vi "PutBool.vi"(8 "error in (no error)":errorcluster, 10 "Boolean":bool, 11 "MsgPackSerializer in":refnum<class "MsgPackSerializer.lvclass">) -> (0 "error out":errorcluster, 3 "MsgPackSerializer out":refnum<class "MsgPackSerializer.lvclass">)   [LabVIEW 2015, in "MsgPackSerializer.lvclass"]
uses:
  MsgPackSerializer.lvclass
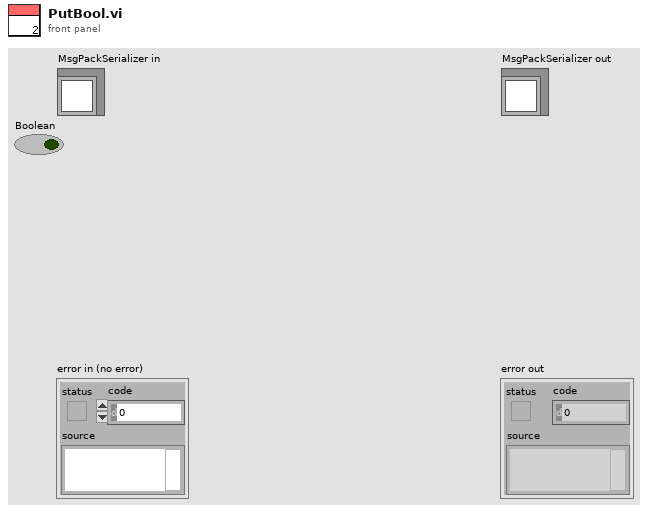
[diagram p1: front panel]
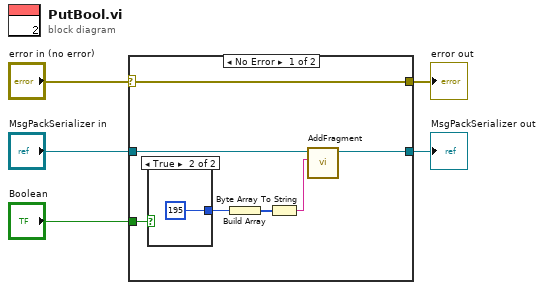
[diagram p0: block diagram]
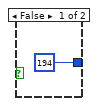
[diagram p2: hidden frame]
diagram:
  n1 = case shown="No Error" "error in (no error)" {
    selector: "error in (no error)" -> [w12 w16]
    tunnel: [w12 w16] -> w4
    tunnel: [w10 w15] -> w2
    tunnel: "MsgPackSerializer in" -> [w11 w15]
    tunnel: "Boolean" -> [w9 _]
    frame No Error {
      n2 = case shown="True" w9 {
        tunnel: [u8 194 ("Number") u8 195 ("Number")] -> w8
        frame False {
        }
        frame True {
        }
      }
      n3 = Build Array(w8) -> (w7:u8[])
      n4 = Byte Array To String(unsigned byte array=w7) -> (string=w6:string)
      n5 = call "AddFragment.vi"("Fragment"=w6, "MsgPackSerializer in"=w11) -> ("MsgPackSerializer out"=w10:refnum<class "MsgPackSerializer.lvclass">)  [unwired: 8 in, 1 out]
    }
    frame Error {
    }
  }
  "error out" <- w4
  "MsgPackSerializer out" <- w2
